vi "wybierz 2 przebiegi do wyswietlenia.vi"(7 "Array in":string[](array[string]), 8 "error in (no error)":errorcluster, 10 "Przebiegi Wfm":waveform(dbl)[](array[waveform])) -> (0 "error out":errorcluster, 2 "Array out":waveform(dbl)[](array[waveform]))   [LabVIEW 2014]
doc: "Wybiera dwa przebiegi wskazane przez comb box do wyœwietlenia"
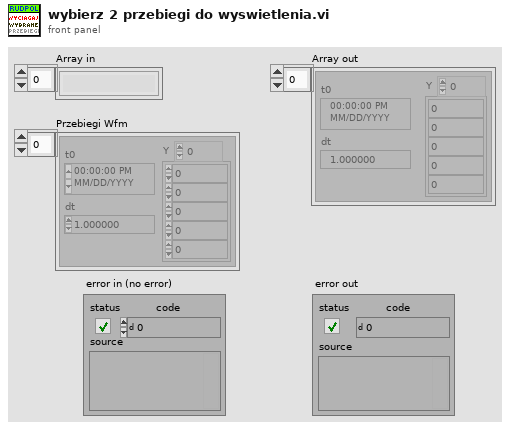
[diagram p1: front panel]
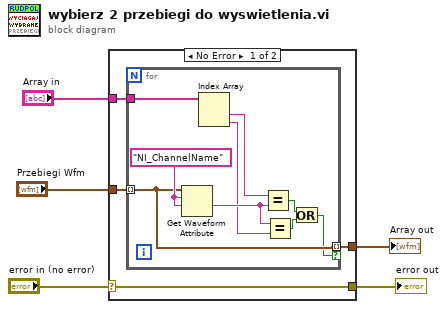
[diagram p0: block diagram]
diagram:
  n1 = case shown="No Error" "error in (no error)" {
    selector: "error in (no error)" -> [w6 w19]
    tunnel: [w9 w20] -> w5
    tunnel: "Array in" -> [w8 _]
    tunnel: "Przebiegi Wfm" -> [w7 w20]
    tunnel: [w6 w19] -> w1
    frame No Error {
      n2 = for {
        tunnel: w7 -> [w17] mode=indexing
        tunnel: w8 -> [w16]
        tunnel: [w17] -> w9 mode=indexing if=w10
        w18 = "NI_ChannelName" ("name")
        n3 = Get Waveform Attribute(5:w18, 6:w18, 7:w17) -> (1:w14:string)  [unwired: 1 in, 3 out]
        n4 = Index Array(array=w16) -> (element #1=w15:string, element #2=w13:string)  [unwired: 2 in]
        n5 = Equal?(x=w15, y=w14) -> (x = y?=w11:bool)
        n6 = Equal?(x=w14, y=w13) -> (x = y?=w12:bool)
        n7 = Or(x=w11, y=w12) -> (x .or. y?=w10:bool)
      }
    }
    frame Error {
    }
  }
  "Array out" <- w5
  "error out" <- w1
